vi "MB MFC Valve Override+.vi"(7 "Action":T2, 8 "error in (no error)":errorcluster, 9 "Override":T1, 11 "TCP Ref":refnum<k5>) -> (0 "error out":errorcluster, 1 "Override":T1, 3 "dup TCP Ref":refnum<k5>)   [LabVIEW 2011]
doc: "This VI reads or writes the valve override of an MKS Modbus MFC. If it was set, then the VI reads the override to make sure it was properly set."
uses:
  Type Definitions/Modbus Action.ctl
  Type Definitions/Valve Override.ctl
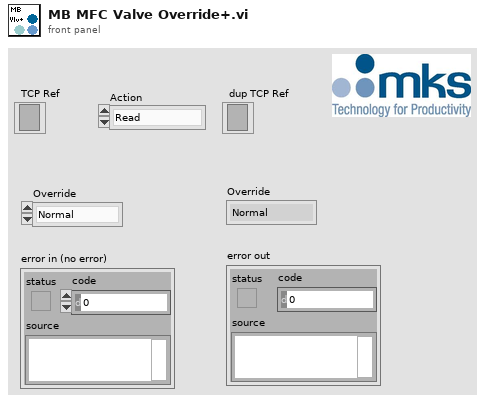
[diagram p1: front panel]
types:
  T1 = typedef "Valve Override.ctl" = enum16{"Normal", "Close", "Open"}
  T2 = typedef "Modbus Action.ctl" = enum16{"Read", "Write"}
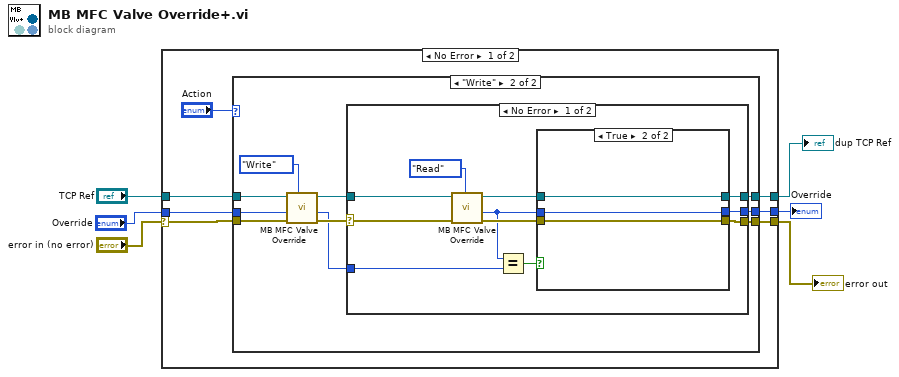
[diagram p0: block diagram]
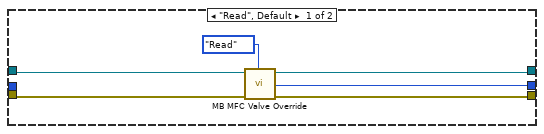
[diagram p2: hidden frame]
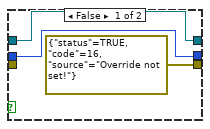
[diagram p3: hidden frame]
diagram:
  n1 = case shown="No Error" "error in (no error)" {
    selector: "error in (no error)" -> [w12 w51]
    tunnel: "TCP Ref" -> [w13 w52]
    tunnel: [w11 w52] -> w4
    tunnel: [w10 w51] -> w3
    tunnel: [w9 w50] -> w1
    tunnel: "Override" -> [w7 w50]
    frame No Error {
      n2 = case shown="\"Write\"" "Action" {
        tunnel: w13 -> [w14 w29]
        tunnel: w12 -> [w18 w26]
        tunnel: [w15 w23] -> w11
        tunnel: [w17 w22] -> w10
        tunnel: [w16 w21] -> w9
        tunnel: w7 -> [_ w20]
        frame "Read", Default {
          n3 = call "MB MFC Valve Override.vi"("Action"=Modbus_Action."Read", "error in (no error)"=w18, "TCP Ref"=w14) -> ("error out"=w17:errorcluster, "Override"=w16:T1, "dup TCP Ref"=w15:refnum<k5>)  [unwired: 6 in]
        }
        frame "Write" {
          n4 = call "MB MFC Valve Override.vi"("Action"=Modbus_Action."Write", "error in (no error)"=w26, "Override"=w20, "TCP Ref"=w29) -> ("error out"=w25:errorcluster, "Override"=w24:T1, "dup TCP Ref"=w28:refnum<k5>)  [unwired: 5 in]
          n5 = case shown="No Error" w25 {
            selector: w25 -> [w38 w48]
            tunnel: w28 -> [w40 w47]
            tunnel: w24 -> [w30 w49]
            tunnel: [w36 w47] -> w23
            tunnel: [w35 w48] -> w22
            tunnel: [w33 w49] -> w21
            frame No Error {
              n6 = call "MB MFC Valve Override.vi"("Action"=Modbus_Action."Read", "error in (no error)"=w38, "TCP Ref"=w40) -> ("error out"=w34:errorcluster, "Override"=w31:T1, "dup TCP Ref"=w37:refnum<k5>)  [unwired: 6 in]
              n7 = Equal?(x=w31, y=w30) -> (x = y?=w32:bool)
              n8 = case shown="True" w32 {
                tunnel: [w42 w46] -> w36
                tunnel: w37 -> [w42 w46]
                tunnel: [errorcluster {"status"=TRUE, "code"=16, "source"="Override not set!"} ("error out") w45] -> w35
                tunnel: w34 -> [_ w45]
                tunnel: [w41 w44] -> w33
                tunnel: w31 -> [w41 w44]
                frame False {
                }
                frame True {
                }
              }
            }
            frame Error {
            }
          }
        }
      }
    }
    frame Error {
    }
  }
  "dup TCP Ref" <- w4
  "error out" <- w3
  "Override" <- w1
